vi "Special Time  UPH.vi"(8 "error in (no error)":errorcluster) -> (0 "error out":errorcluster)   [LabVIEW 2014]
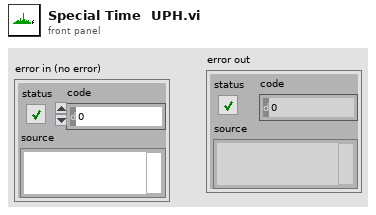
[diagram p1: front panel]
types:
  T1 = typedef "FTT Display Type.ctl" = cluster{"Line.No":string, "Model":string, "Color":string, "UPH":dbl, "Plan":dbl, "Target Rate":dbl, "Target ":dbl, "Actual":dbl, "FTT":dbl, "FTT Rate":dbl, "Repaired":dbl, "Reject":dbl, "Ouline":dbl, "Line State":string}
  T2 = cluster{"Display":T1, "Class":enum16{"Big", "Small"}}
  T3 = typedef "UPH Config.ctl" = cluster{"Line_No":string, "Model":string, "B_UPH ":i16, "S_UPH  ":i16, "Class":enum16{"Big", "Small"}}
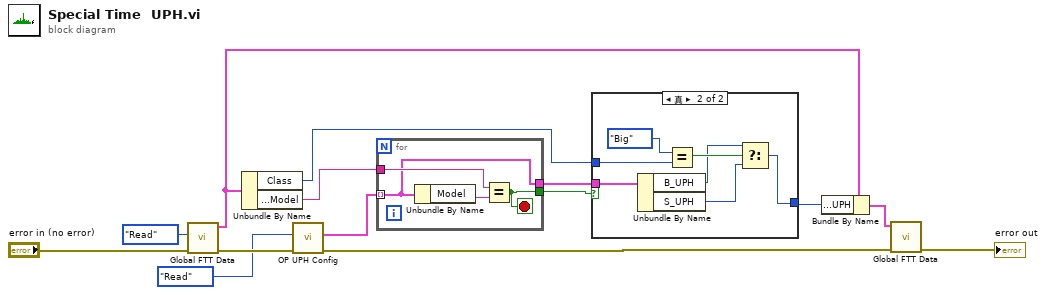
[diagram p0: block diagram]
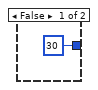
[diagram p2: hidden frame]
diagram:
  n1 = call "Global FTT Data.vi"("error in (no error)"="error in (no error)", "Mode"=enum16{"Read", "Write"}."Read") -> ("error out"=w11:errorcluster, "Cluster"=w4:T2)  [unwired: 8 in]
  n2 = Unbundle By Name(w4) -> ("Class"=w8:enum16{"Big", "Small"}, "Display.Model"=w9:string)
  n3 = call "OP UPH Config.vi"("error in (no error)"=w11, "Enum"=enum16{"init", "Read", "Write"}."Read") -> ("error out"=w7:errorcluster, "UPH out"=w10:T3[])  [unwired: 7 in, 1 out]
  n4 = for {
    tunnel: w10 -> [w16] mode=indexing
    tunnel: w9 -> [w17]
    tunnel: [w16] -> w12
    tunnel: [w15] -> w1
    stop <- w15 stop-if-true
    n5 = Unbundle By Name(w16) -> ("Model"=w18:string)
    n6 = Equal?(x=w17, y=w18) -> (x = y?=w15:bool)
  }
  n7 = case shown="真" w1 {
    tunnel: w8 -> [_ w24]
    tunnel: w12 -> [_ w26]
    tunnel: [i16 30 ("UPH") w20] -> w3
    frame False {
    }
    frame True {
      n8 = Unbundle By Name(w26) -> ("B_UPH"=w22:i16, "S_UPH"=w21:i16)
      n9 = Equal?(x=enum16{"Big", "Small"}."Big" ("Class"), y=w24) -> (x = y?=w23:bool)
      n10 = Select(t=w22, s=w23, f=w21) -> (s? t:f=w20:i16)
    }
  }
  n11 = Bundle By Name(cluster=w4, "Display.UPH"=w3) -> (w2:T2)
  n12 = call "Global FTT Data.vi"("error in (no error)"=w7, "Display"=w2) -> ("error out"=→"error out":errorcluster)  [unwired: 8 in, 1 out]
